vi "Cleanup_Robotics_Cape.vi"(8 "error in (no error)":errorcluster) -> (0 "error out":errorcluster, 3 "Stop Local Variabl":bool)   [LabVIEW 2014]
uses:
  <userlib>/UCSD Robotics Lab/Robotics-Cape/LV/libroboticscape.lvlib
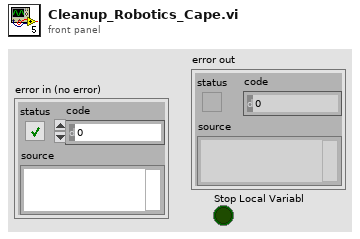
[diagram p1: front panel]
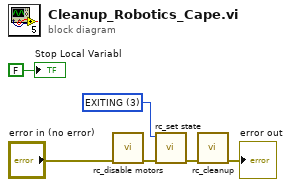
[diagram p0: block diagram]
diagram:
  w4 = u32 3 items=["UNINITIALIZED", "RUNNING", "PAUSED", "EXITING"] ("new_state")
  n1 = call <userlib>:"rc_disable motors.vi"("error in (no error)"="error in (no error)") -> ("error out"=w2:errorcluster)  [unwired: 9 in, 1 out]
  n2 = call <userlib>:"rc_set state.vi"("error in (no error)"=w2, "new_state"=w4) -> ("error out"=w3:errorcluster)  [unwired: 8 in, 1 out]
  n3 = call <userlib>:"rc_cleanup.vi"("error in (no error)"=w3) -> ("error out"=→"error out":errorcluster)  [unwired: 9 in, 1 out]
  "Stop Local Variabl" <- FALSE ("Boolean")
